vi "TEST - Scan Variant from String.vi"(8 "error in (no error)":errorcluster) -> (0 "error out":errorcluster, 2 "Pass":bool)   [LabVIEW 2009]
panel:
  out "Failures":T1(array[cluster])
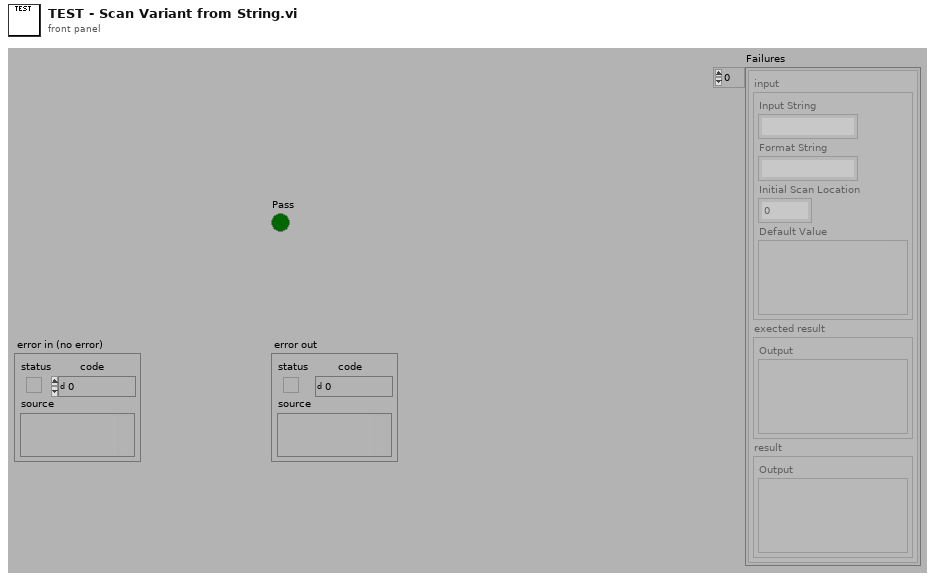
[diagram p1: front panel]
types:
  T1 = cluster{"input":cluster{"Input String":string, "Format String":string, "Initial Scan Location":u32, "Default Value":variant}, "exected result":cluster{"Output":variant}, "result":cluster{"Output":variant}}[]
  T2 = cluster{"input":cluster{"Input String":string, "Format String":string, "Initial Scan Location":u32, "Default Value":variant}, "exected result":cluster{"Output":variant}, "result":cluster{"Output":variant}}
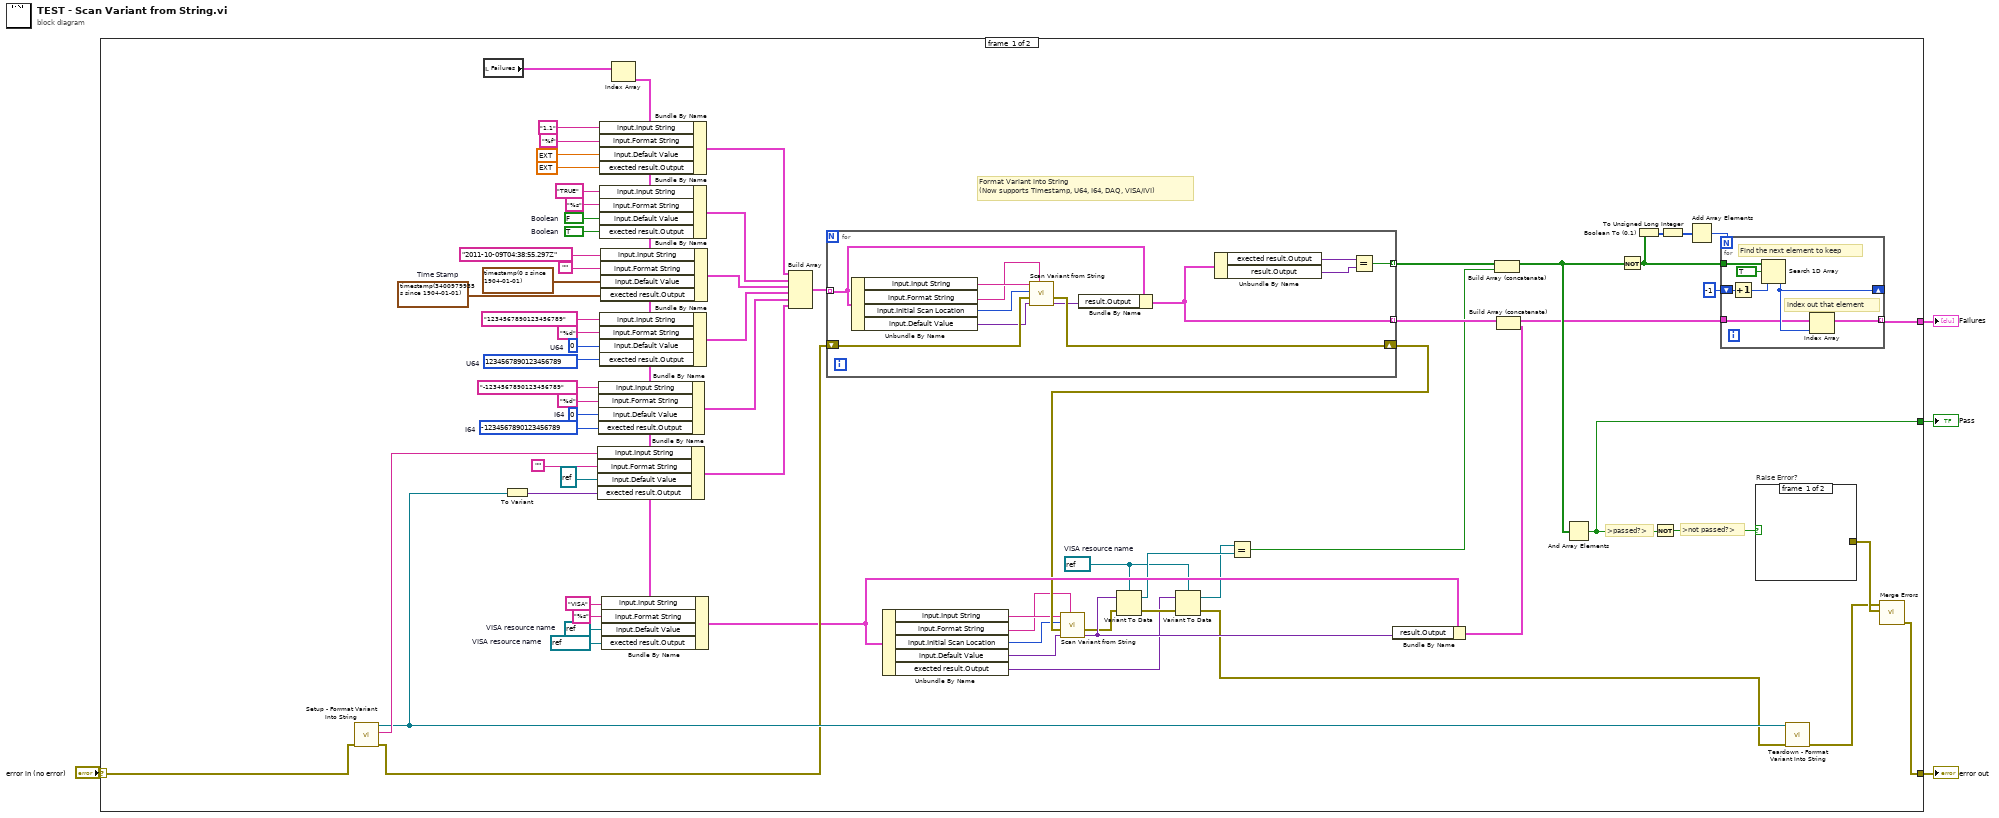
[diagram p0: block diagram]
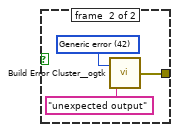
[diagram p2: hidden frame]
diagram:
  n1 = case shown="No Error" "error in (no error)" {
    selector: "error in (no error)" -> [w36 w98]
    tunnel: [w64 _] -> w4
    tunnel: [w75 w98] -> w2
    tunnel: [w67 _] -> w1
    frame #0 {
      w9 = refnum<visa-resource-name> refnum  # VISA resource name
      w5 = refnum<visa-resource-name> "VISA"  # VISA resource name
      w6 = refnum<visa-resource-name> refnum  # VISA resource name
      w45 = u64 0  # U64
      w46 = i64 0  # I64
      w56 = timestamp(3400979935.297 s since 1904-01-01)  # Time Stamp
      w48 = i64 -1234567890123456789  # I64
      w50 = u64 1234567890123456789  # U64
      w59 = TRUE  # Boolean
      w60 = FALSE  # Boolean
      # "Format Variant into String\n(Now supports Timestamp, U64, I64, DAQ, VISA/IVI)"
      # ">not passed?>"
      # ">passed?>"
      n2 = call "Setup - Forrmat Variant Into String.vi"("error in (no error)"=w36) -> ("error out"=w30:errorcluster, "Input String"=w39:string, "Refnum"=w37:refnum<file>)  [unwired: 8 in]
      n3 = local read "Failures"() -> (w66:T1)
      n4 = To Variant(anything=w37) -> (Variant=w43:variant)
      n5 = Index Array(array=w66) -> (element=w27:T2)  [unwired: 1 in]
      n6 = Bundle By Name(cluster=w27, "input.Input String"=w39, "input.Format String"="", "input.Default Value"=refnum<file> refnum ("refnum out"), "exected result.Output"=w43) -> (w40:T2)
      n7 = Bundle By Name(cluster=w27, "input.Input String"="-1234567890123456789" ("y"), "input.Format String"="%d" ("format string"), "input.Default Value"=w46, "exected result.Output"=w48) -> (w44:T2)
      n8 = Bundle By Name(cluster=w27, "input.Input String"="1.1" ("Input String"), "input.Format String"="%f" ("Format String (optional)"), "input.Default Value"=ext 0.0, "exected result.Output"=ext 1.1) -> (w31:T2)
      n9 = Bundle By Name(cluster=w27, "input.Input String"="TRUE" ("y"), "input.Format String"="%s" ("format string"), "input.Default Value"=w60, "exected result.Output"=w59) -> (w61:T2)
      n10 = Bundle By Name(cluster=w27, "input.Input String"="1234567890123456789" ("y"), "input.Format String"="%d" ("format string"), "input.Default Value"=w45, "exected result.Output"=w50) -> (w54:T2)
      n11 = Bundle By Name(cluster=w27, "input.Input String"="2011-10-09T04:38:55.297Z" ("y"), "input.Format String"="", "input.Default Value"=timestamp(0 s since 1904-01-01) ("Time Stamp"), "exected result.Output"=w56) -> (w63:T2)
      n12 = Bundle By Name(cluster=w27, "input.Input String"="VISA" ("y"), "input.Format String"="%s" ("format string"), "input.Default Value"=w6, "exected result.Output"=w5) -> (w26:T2)
      n13 = Build Array(w31, w61, w63, w54, w44, w40) -> (w53:T1)
      n14 = for {
        tunnel: w53 -> [w94] mode=indexing
        shift-right: [w84] -> w25
        shift-left: w30 -> [w86]
        tunnel: [w93] -> w22 mode=indexing
        tunnel: [w90] -> w20 mode=indexing
        n15 = Unbundle By Name(w94) -> ("input.Input String"=w89:string, "input.Format String"=w88:string, "input.Initial Scan Location"=w87:u32, "input.Default Value"=w85:variant)
        n16 = call "Scan Variant from String.vi"("Format String (optional)"=w88, "Default Value"=w85, "error in (no error)"=w86, "Initial Scan Location"=w87, "Input String"=w89) -> ("Output"=w83:variant, "error out"=w84:errorcluster)  [unwired: 3 in, 2 out]
        n17 = Bundle By Name(cluster=w94, "result.Output"=w83) -> (w90:T2)
        n18 = Unbundle By Name(w90) -> ("exected result.Output"=w92:variant, "result.Output"=w91:variant)
        n19 = Equal?(x=w92, y=w91) -> (x = y?=w93:bool)
      }
      n20 = Unbundle By Name(w26) -> ("input.Input String"=w19:string, "input.Format String"=w18:string, "input.Initial Scan Location"=w17:u32, "input.Default Value"=w16:variant, "exected result.Output"=w8:variant)
      n21 = call "Scan Variant from String.vi"("Format String (optional)"=w18, "Default Value"=w16, "error in (no error)"=w25, "Initial Scan Location"=w17, "Input String"=w19) -> ("Output"=w15:variant, "error out"=w14:errorcluster)  [unwired: 3 in, 2 out]
      n22 = Variant To Data(error in=w14, Variant=w15, type=w9) -> (error out=w11:errorcluster, data=w13:refnum<visa-resource-name>)
      n23 = Variant To Data(error in=w11, Variant=w8, type=w9) -> (error out=w10:errorcluster, data=w7:refnum<visa-resource-name>)
      n24 = Equal?(x=w7, y=w13) -> (x = y?=w12:bool)
      n25 = Bundle By Name(cluster=w26, "result.Output"=w15) -> (w24:T2)
      n26 = Build Array (concatenate)(w22, w12) -> (w23:bool[])
      n27 = Build Array (concatenate)(w20, w24) -> (w21:T1)
      n28 = And Array Elements(Boolean array=w23) -> (logical AND=w64:bool)
      n29 = Not(x=w23) -> (.not. x?=w69:bool[])
      n30 = Boolean To (0,1)(Boolean=w69) -> (0, 1=w70:i16[])
      n31 = Not(x=w64) -> (.not. x?=w73:bool)
      n32 = To Unsigned Long Integer(number=w70) -> (unsigned 32bit integer=w68:u32[])
      n33 = Add Array Elements(numeric array=w68) -> (sum=w71:u32)
      n34 = for {
        N: w71 -> [_]
        tunnel: w21 -> [w78]
        tunnel: w69 -> [w82]
        shift-right: [w79] -> _
        shift-left: -1 ("start index (0)") -> [w80]
        tunnel: [w77] -> w67 mode=indexing
        # "index out that element"
        # "Find the next element to keep"
        n35 = Increment(x=w80) -> (x+1=w76:i32)
        n36 = Search 1D Array(1D array=w82, element=TRUE, start index (0)=w76) -> (index of element=w79:i32)
        n37 = Index Array(array=w78, index=w79) -> (element=w77:T2)
      }
      n38 = case "Raise Error?" shown="True" w73 {
        tunnel: [_ w95] -> w74
        frame #0 {
        }
        frame #1 {
          w96 = 42 items=["No error", "Argument error", "Memory is full", "Out of zone", "End of file", "File already open", "Generic file I/O error", "File not found", "File permission error", "Disk is full", "Duplicate path", "Too many files open", "System feature not enabled", "Resource file not found", "Cannot add resource", "Resource not found", "Image not found", "Image memory error", "Pen does not exist", "Config type invalid", "Config token not found", "Config parse error", "Config memory error", "Bad external code format", "Bad external code offset", "External code not present", "Null window", "Destroy window error", "Null menu", "Print aborted", "Bad print record", "Print driver error", "Windows error during printing", "Memory error during printing", "Print dialog error", "Generic print error", "Invalid device refnum", "Device not found", "Device parameter error", "Device unit error", "Cannot open device", "Device call aborted", "Generic error", "Cancelled by user", "Object ID too low", "Object ID too high", "Object not in heap", "Unknown heap", "Unknown object (invalid DefProc)", "Unknown object (DefProc not in table)", "Message out of range", "Invalid (null) method", "Unknown message", "Manager call not supported", "Bad address", "Network operation in progress", "Network operation timed out", "Connection is busy", "Network attribute not supported", "Network error", "Address in use", "System out of memory", "Connection aborted", "Connection refused", "Not connected", "Already connected", "Connection closed", "Initialization error (interapplication manager)", "Bad occurrence", "Wait on unbound occurrence handler", "Occurrence queue overflow", "Datalog type conflict", "Unused", "Unrecognized type (interapplication manager)", "Memory corrupt", "Failed to make temporary DLL", "Old CIN version", "Drag socket not found", "Failed to load drop-object", "Failed to register OLE object", "Failed to release OLE object", "Format specifier type mismatch", "Unknown format specifier", "Too few format specifiers", "Too many format specifiers", "Scan failed", "Newer CIN version", "Error converting to variant", "Runtime menu error", "Password tampered", "Variant attribute not found", "Incompatible variant data type", "Event data is not available", "Event Store is not present", "Occurrence is not found", "Event Queue is not created", "Event info is not available", "Refnum passed is NULL", "Error retrieving Class GUID", "Error retrieving CoClass GUID", "Error retrieving TypeLib GUID.", "Bad built application magic bytes.", "Specific driver is different from the specific driver associated with the Logical Name.", "There is no session opened to the class driver.", "Max Error", "MAX - Error with config objects", "MAX - Error loading configuration", "MAX - Group not supported"]
          n39 = call <userlib>:"Build Error Cluster__ogtk.vi"("String to Prepend to source (\"\")"="unexpected output" ("String to Prepend to source (\"\")"), "code"=w96) -> ("error out"=w95:errorcluster)
        }
      }
      n40 = call "Teardown - Forrmat Variant Into String.vi"("error in (no error)"=w10, "Refnum"=w37) -> ("error out"=w38:errorcluster)  [unwired: 9 in]
      n41 = call <vilib>:"Merge Errors.vi"("error in 2 (no error)"=w74, "error in 1 (no error)"=w38) -> ("error out"=w75:errorcluster)  [unwired: 5 in]
    }
    frame #1 {
    }
  }
  "Pass" <- w4
  "error out" <- w2
  "Failures" <- w1
